vi "Read pin_name.vi"(8 "error in (no error)":errorcluster, 11 "DMM_Base in":refnum<class "DMM_Base.lvclass">) -> (0 "error out":errorcluster, 2 "pin_name":string, 3 "DMM_Base out":refnum<class "DMM_Base.lvclass">)   [LabVIEW 2021, in "DMM_Base.lvclass"]
uses:
  DMM_Base.lvclass
  DMM_Base.lvclass/DMM_Base.ctl
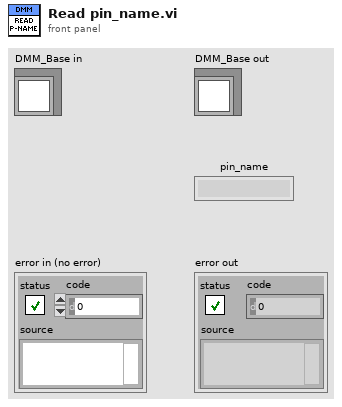
[diagram p1: front panel]
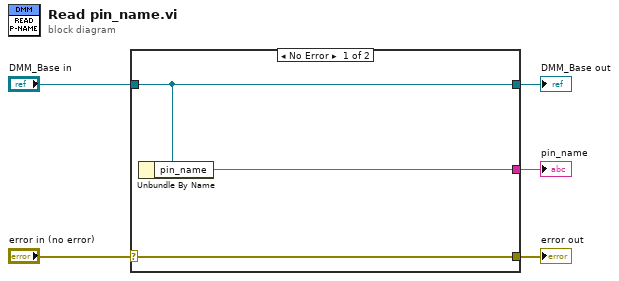
[diagram p0: block diagram]
diagram:
  n1 = case shown="No Error" "error in (no error)" {
    selector: "error in (no error)" -> [w8 w9]
    tunnel: [w8 w9] -> w4
    tunnel: [w7 w10] -> w2
    tunnel: "DMM_Base in" -> [w7 w10]
    tunnel: [w6 _] -> w1
    frame No Error {
      n2 = Unbundle By Name(w7) -> ("pin_name"=w6:string)
    }
    frame Error {
    }
  }
  "error out" <- w4
  "DMM_Base out" <- w2
  "pin_name" <- w1
